vi "Mandelbrot V1.vi"() -> ()   [LabVIEW 2011]
panel:
  out "XY Graph":cluster{i32, i32}[](graph)
  out "Duration (S)":dbl
  out "End Time":timestamp
  out "Start Time":timestamp
  out "C":cdb
  out "Intensity Graph":i32[][](graph)
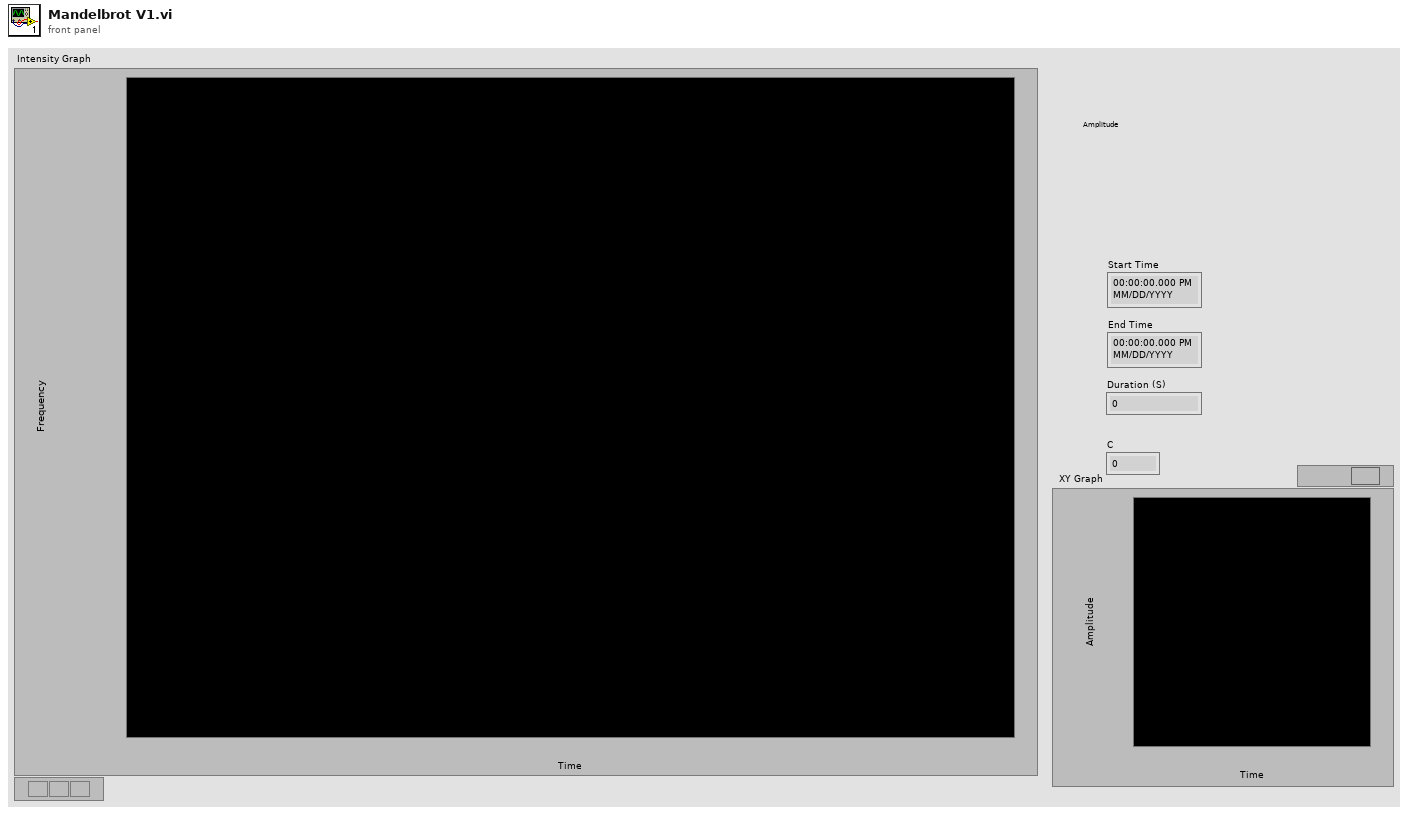
[diagram p1: front panel]
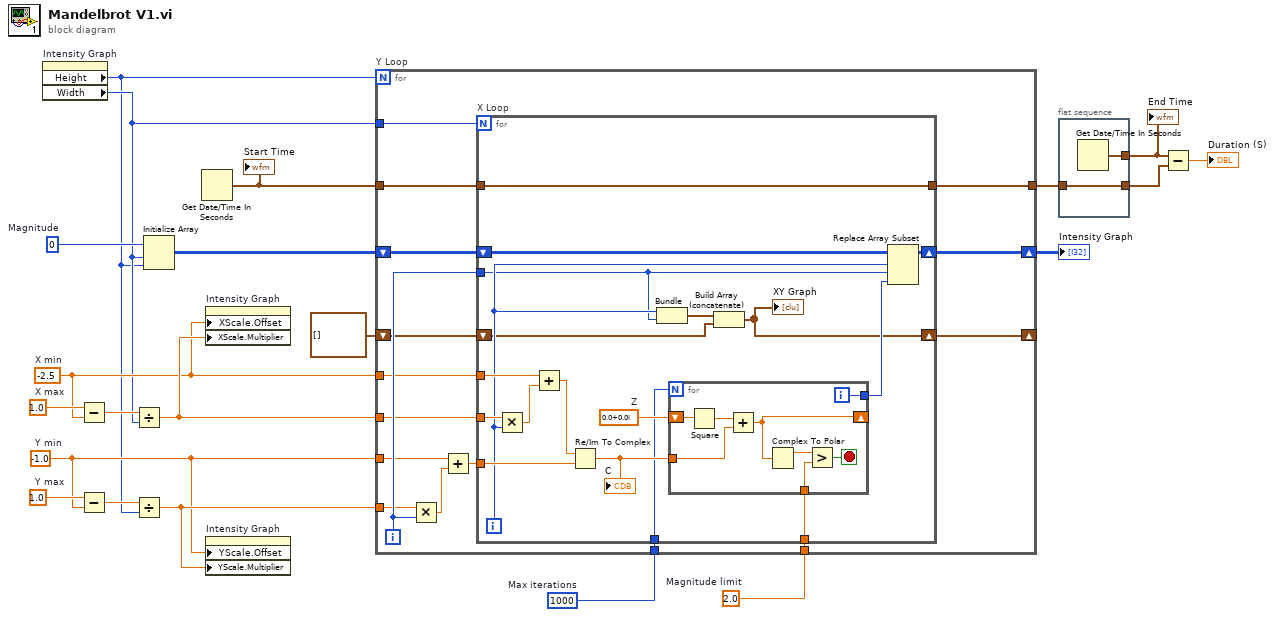
[diagram p0: block diagram]
diagram:
  w10 = 2.0  # Magnitude limit
  w11 = 1000  # Max iterations
  w12 = -1.0  # Y min
  w14 = 1.0  # Y max
  w20 = 0  # Magnitude
  w16 = -2.5  # X min
  w18 = 1.0  # X max
  n1 = property on="Intensity Graph" class="IntGraph (strict)"() -> ("Height"=w3:u32, "Width"=w4:u32)  [unwired: 2 in, 2 out]
  n2 = Subtract(x=w18, y=w16) -> (x-y=w21:dbl)
  n3 = Subtract(x=w14, y=w12) -> (x-y=w15:dbl)
  n4 = Divide(x=w21, y=w4) -> (x/y=w17:dbl)
  n5 = Divide(x=w15, y=w3) -> (x/y=w13:dbl)
  n6 = Initialize Array(w20, w4, w3) -> (w19:i32[][])
  n7 = Get Date/Time In Seconds() -> (seconds since 1Jan1904=w9:timestamp)
  "Start Time" <- w9
  n8 = property on="Intensity Graph" class="IntGraph (strict)"("XScale.Offset"=w16, "XScale.Multiplier"=w17) -> ()  [unwired: 2 in, 2 out]
  n9 = property on="Intensity Graph" class="IntGraph (strict)"("YScale.Offset"=w12, "YScale.Multiplier"=w13) -> ()  [unwired: 2 in, 2 out]
  n10 = for "Y Loop" {
    N: w3 -> [_]
    tunnel: w17 -> [w30]
    tunnel: w16 -> [w32]
    shift-right: [w24] -> w2
    shift-left: w19 -> [w35]
    tunnel: w12 -> [w33]
    tunnel: w13 -> [w31]
    tunnel: w11 -> [w29]
    tunnel: w10 -> [w28]
    tunnel: w4 -> [w27]
    tunnel: w9 -> [w26]
    tunnel: [w25] -> w8
    shift-right: [w23] -> _
    shift-left: cluster{i32, i32}[] [] -> [w22]
    i -> [w34]
    n11 = Multiply(x=w31, y=w34) -> (x*y=w37:dbl)
    n12 = Add(x=w33, y=w37) -> (x+y=w36:dbl)
    n13 = for "X Loop" {
      N: w27 -> [_]
      tunnel: w30 -> [w53]
      tunnel: w36 -> [w54]
      tunnel: w32 -> [w52]
      shift-right: [w48] -> w24
      shift-left: w35 -> [w49]
      tunnel: w34 -> [w41]
      tunnel: w29 -> [w46]
      tunnel: w28 -> [w45]
      tunnel: w26 -> [w44]
      tunnel: [w44] -> w25
      shift-right: [w39] -> w23
      shift-left: w22 -> [w38]
      i -> [w42]
      w47 = cdb 0.0+0.0i  # Z
      n14 = Multiply(x=w53, y=w42) -> (x*y=w55:dbl)
      n15 = Add(x=w52, y=w55) -> (x+y=w51:dbl)
      n16 = Re/Im To Complex(1:w54, 2:w51) -> (0:w50:cdb)
      "C" <- w50
      n17 = Bundle(w42, w41) -> (w40:cluster{i32, i32})  [unwired: 1 in]
      n18 = for {
        N: w46 -> [_]
        tunnel: w50 -> [w62]
        shift-right: [w60] -> _
        shift-left: w47 -> [w63]
        tunnel: w45 -> [w58]
        tunnel: [w56] -> w43
        i -> [w56]
        stop <- w57 stop-if-true
        n19 = Square(x=w63) -> (x^2=w61:cdb)
        n20 = Add(x=w61, y=w62) -> (x+y=w60:cdb)
        n21 = Complex To Polar(r * e^(i*theta)=w60) -> (r=w59:dbl)  [unwired: 1 out]
        n22 = Greater?(x=w59, y=w58) -> (0:w57:bool)
      }
      n23 = Build Array (concatenate)(w40, w38) -> (w39:cluster{i32, i32}[])
      "XY Graph" <- w39
      n24 = Replace Array Subset(array=w49, new element=w43, index (row)=w42, index (col)=w41) -> (w48:i32[][])
    }
  }
  "Intensity Graph" <- w2
  n25 = flat-sequence {
    tunnel: w8 -> [w64]
    tunnel: [w65] -> w6
    tunnel: [w64] -> w7
    frame #0 {
      n26 = Get Date/Time In Seconds() -> (seconds since 1Jan1904=w65:timestamp)
    }
  }
  n27 = Subtract(x=w6, y=w7) -> (x-y=→"Duration (S)":dbl)
  "End Time" <- w6
